vi "Bundle by position.vi"() -> ()   [LabVIEW 2015]
panel:
  in  "VI Refnum":refnum<vi>
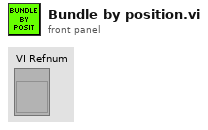
[diagram p1: front panel]
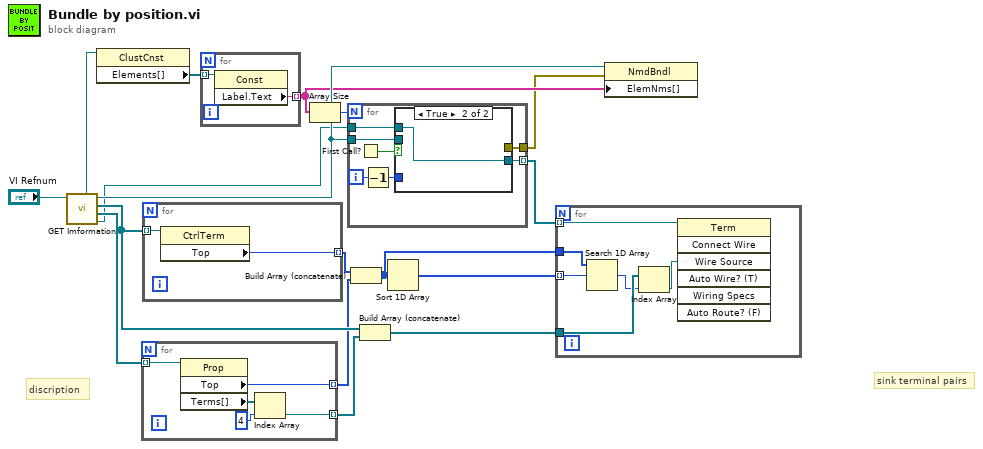
[diagram p0: block diagram]
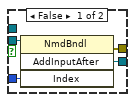
[diagram p2: hidden frame]
diagram:
  # "discription"
  # "sink terminal pairs"
  n1 = call "GET Imformation.vi"("VI Refnum"="VI Refnum") -> ("Term Refnum"=w2:refnum<vi>, "Property Reference"=w11:refnum<vi>[], "Terms Reference"=w15:refnum<vi>[], "Bundle Reference"=w5:refnum<vi>, "Cluster Constant reference"=w8:refnum<vi>)  [unwired: 6 in]
  n2 = property class="ClustCnst"(reference=w8) -> ("Elements[]"=w7:refnum<vi>[])  [unwired: 1 in, 2 out]
  n3 = for {
    tunnel: w11 -> [w20] mode=indexing
    tunnel: [w19] -> w10 mode=indexing
    tunnel: [w18] -> w9 mode=indexing
    n4 = property class="Prop"(reference=w20) -> ("Top"=w18:i32, "Terms[]"=w22:refnum<vi>[])  [unwired: 1 in, 2 out]
    n5 = Index Array(array=w22, index=4) -> (element=w19:refnum<vi>)
  }
  n6 = for {
    tunnel: w15 -> [w24] mode=indexing
    tunnel: [w23] -> w16 mode=indexing
    n7 = property class="CtrlTerm"(reference=w24) -> ("Top"=w23:i32)  [unwired: 1 in, 2 out]
  }
  n8 = for {
    tunnel: w7 -> [w26] mode=indexing
    tunnel: [w25] -> w3 mode=indexing
    n9 = property class="Const"(reference=w26) -> ("Label.Text"=w25:string)  [unwired: 1 in, 2 out]
  }
  n10 = Array Size(array=w3) -> (size(s)=w6:i32)
  n11 = for {
    N: w6 -> [_]
    tunnel: w5 -> [w33]
    tunnel: w2 -> [w32]
    tunnel: [w28] -> w4 mode=indexing
    tunnel: [w27] -> w1
    i -> [w30]
    n12 = First Call?() -> (First Call?: T/F=w31:bool)
    n13 = Decrement(x=w30) -> (x-1=w29:i32)
    n14 = case shown="True" w31 {
      tunnel: w33 -> [w37 _]
      tunnel: w29 -> [w36 _]
      tunnel: [w35 w38] -> w28
      tunnel: w32 -> [_ w38]
      tunnel: [w34 _] -> w27
      frame False {
        n15 = invoke class="NmdBndl" method="AddInputAfter"(reference=w37, "Index"=w36) -> (error out=w34:errorcluster, "AddInputAfter"=w35:refnum<vi>)  [unwired: 2 in, 2 out]
      }
      frame True {
      }
    }
  }
  n16 = Build Array (concatenate)(w16, w9) -> (w13:i32[])
  n17 = Build Array (concatenate)(w15, w10) -> (w14:refnum<vi>[])
  n18 = Sort 1D Array(array=w13) -> (sorted array=w12:i32[])
  n19 = for {
    tunnel: w12 -> [w42] mode=indexing
    tunnel: w14 -> [w44]
    tunnel: w13 -> [w43]
    tunnel: w4 -> [w39] mode=indexing
    n20 = Search 1D Array(1D array=w43, element=w42) -> (index of element=w41:i32)  [unwired: 1 in]
    n21 = Index Array(array=w44, index=w41) -> (element=w40:refnum<vi>)
    n22 = invoke class="Term" method="Connect Wire"(reference=w39, "Wire Source"=w40) -> ()  [unwired: 5 in, 7 out]
  }
  n23 = property class="NmdBndl"(reference=w5, error in=w1, "ElemNms[]"=w3) -> ()  [unwired: 2 out]
